vi "Create Handle Click on Graph Msg.vi"(7 "Return Priority (Normal)":T1=enum."Normal", 11 "Return Enqueuer":refnum<class "Message Enqueuer.lvclass">) -> (3 "Handle Click on Graph Msg out":refnum<class "Handle Click on Graph Msg.lvclass">)   [LabVIEW 2020, in "GarphView.lvlib" / "Handle Click on Graph Msg.lvclass"]
uses:
  Handle Click on Graph Msg.lvclass
  Handle Click on Graph Msg.lvclass/Handle Click on Graph Msg.ctl
  <vilib>/gpm_packages/@cs/actor-framework-messages/Source/RoundTripMessage/RoundTripMessage.lvclass
  C:/Program Files (x86)/National Instruments/LabVIEW 2020/vi.lib/gpm_packages/@cs/actor-framework-messages/Source/RoundTripMessage/RoundTripMessage.lvclass
  C:/Program Files (x86)/National Instruments/LabVIEW 2020/vi.lib/ActorFramework/Message/Message.lvclass
  C:/Users/Fred Guo/Desktop/GarphTools/GarphView/GarphView Messages/Handle Click on Graph Msg/Handle Click on Graph Msg.lvclass
  <vilib>/ActorFramework/Message Enqueuer/Message Priority.ctl
  <vilib>/ActorFramework/Message Enqueuer/Message Enqueuer.lvclass
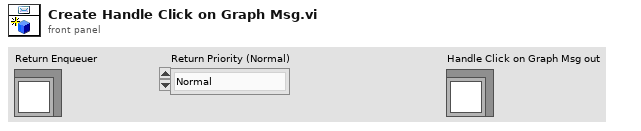
[diagram p1: front panel]
types:
  T1 = typedef "Actor Framework.lvlib/Message Enqueuer.lvclass/Message Priority.ctl" = enum16{"Low", "Normal", "High"}
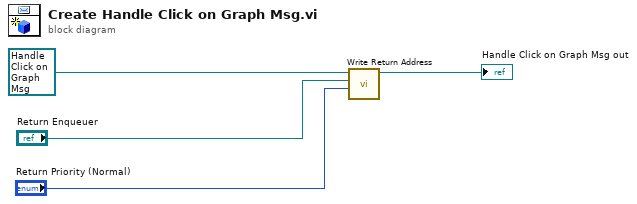
[diagram p0: block diagram]
diagram:
  n1 = call <vilib>:"Write Return Address.vi"("Return Priority (Normal)"="Return Priority (Normal)", "Return Enqueuer"="Return Enqueuer", "RoundTripMessage In"=refnum<class "Handle Click on Graph Msg.lvclass"> refnum ("Handle Click on Graph Msg out")) -> ("RoundTripMessage Out"=→"Handle Click on Graph Msg out":refnum<class "Handle Click on Graph Msg.lvclass">)  [unwired: 8 in]
